vi "Drive Chassies process.vi"(0 "error in":errorcluster) -> ()   [LabVIEW 2012]
uses:
  Or David (Drive Global Data).vi
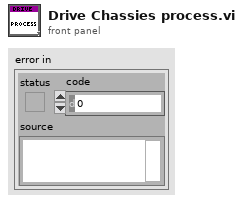
[diagram p1: front panel]
types:
  T1 = typedef "WPI_SolenoidValue.ctl" = enum16{"Off", "On", "Forward", "Reverse"}
  T2 = cluster{"Shifter?":bool, "Axisses":dbl[], "Shifter Value":T1}
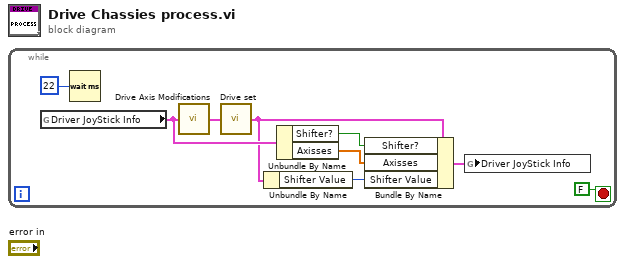
[diagram p0: block diagram]
diagram:
  n1 = while {
    stop <- FALSE stop-if-true
    n2 = global read "Or David (Drive Global Data).vi" "Driver JoyStick Info"() -> (w6:T2)
    n3 = Wait (ms)(milliseconds to wait=u32 22) -> ()  [unwired: 1 out]
    n4 = call "Drive Axis Modifications.vi"("Driver JoyStick Info"=w6) -> ("Driver JoyStick Info Out"=w9:T2)
    n5 = call "Drive set.vi"("Driver JoyStick Info"=w9) -> ("Driver JoyStick Info Out"=w5:T2)
    n6 = Unbundle By Name(w5) -> ("Shifter Value"=w4:T1)
    n7 = Unbundle By Name(w6) -> ("Shifter?"=w3:bool, "Axisses"=w2:dbl[])
    n8 = Bundle By Name(cluster=w5, "Shifter?"=w3, "Axisses"=w2, "Shifter Value"=w4) -> (w1:T2)
    n9 = global write "Or David (Drive Global Data).vi" "Driver JoyStick Info"(w1) -> ()
  }
